vi "EF_ReadIniFile.vi"(11 "Path":path) -> (2 "EF_DAQThread_IniData":T1, 3 "EF_DAQThread_Data":T2)   [LabVIEW 2017]
uses:
  Types/EF_DAQThread_Data.ctl
  _lib/PQ/PicoHarp/PH_InitInfo.ctl
  Types/EF_GUIThread_IniData.ctl
  <vilib>/Utility/config.llb/Read Key (String).vi
  <vilib>/Utility/config.llb/Write Key (String).vi
  <vilib>/Utility/config.llb/Read Key (I32).vi
  <vilib>/Utility/config.llb/Write Key (I32).vi
  <vilib>/Utility/config.llb/Read Key (Double).vi
  <vilib>/Utility/config.llb/Write Key (Double).vi
  <vilib>/Utility/config.llb/Read Key (U32).vi
  <vilib>/Utility/config.llb/Write Key (U32).vi
  <vilib>/Utility/config.llb/NI_LVConfig.lvlib
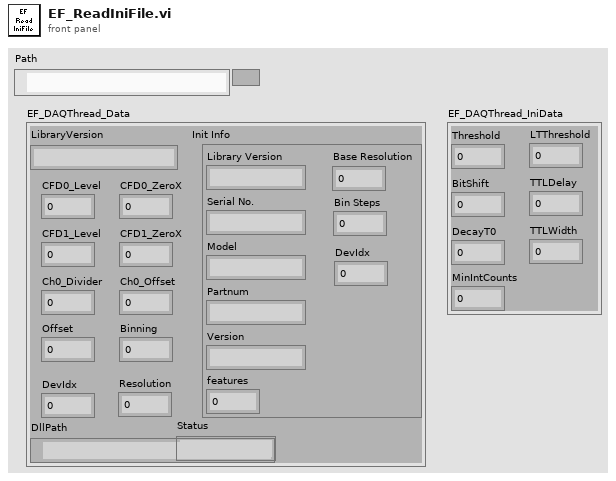
[diagram p1: front panel]
types:
  T1 = typedef "EF_GUIThread_IniData.ctl" = cluster{"Threshold":i32, "BitShift":i32, "DecayT0":dbl, "LTThreshold":dbl, "TTLDelay":i32, "TTLWidth":i32, "MinIntCounts":u32}
  T2 = typedef "EF_DAQThread_Data.ctl" = cluster{"LibraryVersion":string, "CFD0_Level":i32, "CFD0_ZeroX":i32, "CFD1_Level":i32, "CFD1_ZeroX":i32, "Ch0_Divider":i32, "Ch0_Offset":i32, "Init Info":T3, "DevIdx":i32, "Offset":i32, "Binning":i32, "Resolution":dbl, "DllPath":path, "Status":string}
  T3 = typedef "PH_InitInfo.ctl" = cluster{"Library Version":string, "Serial No.":string, "Model":string, "Partnum":string, "Version":string, "features":i32, "Base Resolution":dbl, "Bin Steps":i32, "DevIdx":i32}
  T4 = typedef "NI_LVConfig.lvlib/Config Data RefNum.ctl" = refnum<k1>
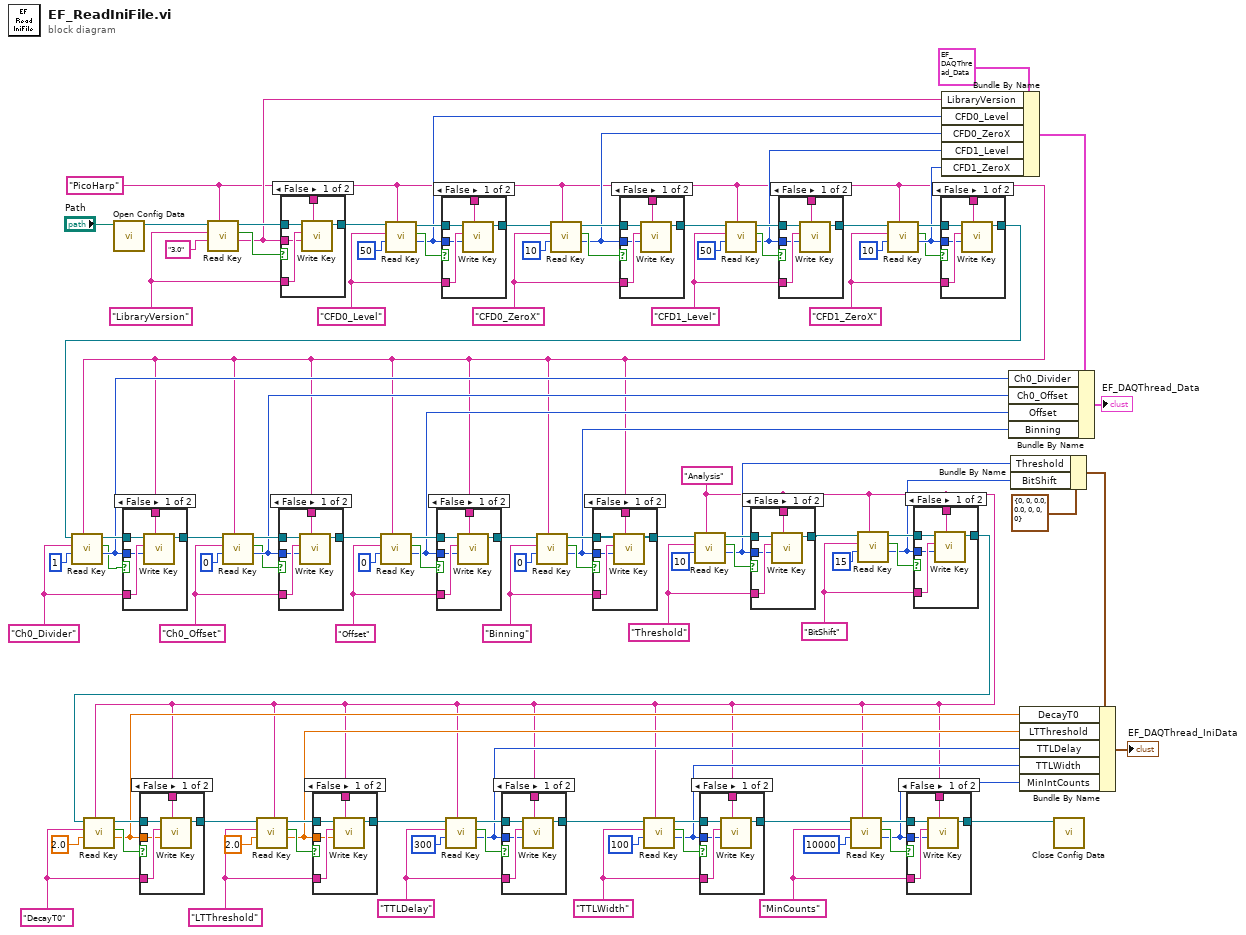
[diagram p0: block diagram]
diagram:
  w8 = "MinCounts" ("key")
  w19 = "TTLWidth" ("key")
  w27 = "TTLDelay" ("key")
  w29 = "LTThreshold" ("key")
  w37 = "DecayT0" ("key")
  w39 = "BitShift" ("key")
  w3 = "Analysis" ("section")
  w44 = "Threshold" ("key")
  w49 = "Binning" ("key")
  w55 = "Offset" ("key")
  w62 = "Ch0_Offset" ("key")
  w69 = "Ch0_Divider" ("key")
  w76 = "CFD1_ZeroX" ("key")
  w80 = "CFD1_Level" ("key")
  w83 = "CFD0_ZeroX" ("key")
  w89 = "CFD0_Level" ("key")
  w94 = "LibraryVersion" ("key")
  w48 = "PicoHarp" ("section")
  n1 = call <vilib>:"Open Config Data.vi"("configuration file path"="Path") -> ("refnum"=w105:T4)  [unwired: 8 in, 2 out]
  n2 = call-poly <vilib>:"Read Key.vi"("section"=w48, "default value"="3.0", "key"=w94, "refnum"=w105) -> ("value"=w93:string, "found?"=w96:bool, "refnum out"=w95:T4)  [unwired: 4 in, 1 out]
  n3 = case shown="False" w96 {
    tunnel: w95 -> [w111 w112]
    tunnel: w48 -> [w110 _]
    tunnel: w94 -> [w109 _]
    tunnel: w93 -> [w108 _]
    tunnel: [w107 w112] -> w92
    frame False {
      n4 = call-poly <vilib>:"Write Key.vi"("section"=w110, "value"=w108, "key"=w109, "refnum"=w111) -> ("refnum out"=w107:T4)  [unwired: 5 in, 2 out]
    }
    frame True {
    }
  }
  n5 = call-poly <vilib>:"Read Key.vi"("section"=w48, "default value"=50, "key"=w89, "refnum"=w92) -> ("value"=w88:i32, "found?"=w90:bool, "refnum out"=w91:T4)  [unwired: 4 in, 1 out]
  n6 = case shown="False" w90 {
    tunnel: w91 -> [w117 w118]
    tunnel: w48 -> [w116 _]
    tunnel: w89 -> [w115 _]
    tunnel: w88 -> [w114 _]
    tunnel: [w113 w118] -> w87
    frame False {
      n7 = call-poly <vilib>:"Write Key.vi"("section"=w116, "value"=w114, "key"=w115, "refnum"=w117) -> ("refnum out"=w113:T4)  [unwired: 5 in, 2 out]
    }
    frame True {
    }
  }
  n8 = call-poly <vilib>:"Read Key.vi"("section"=w48, "default value"=10, "key"=w83, "refnum"=w87) -> ("value"=w84:i32, "found?"=w85:bool, "refnum out"=w86:T4)  [unwired: 4 in, 1 out]
  n9 = case shown="False" w85 {
    tunnel: w86 -> [w123 w124]
    tunnel: w48 -> [w122 _]
    tunnel: w83 -> [w121 _]
    tunnel: w84 -> [w120 _]
    tunnel: [w119 w124] -> w82
    frame False {
      n10 = call-poly <vilib>:"Write Key.vi"("section"=w122, "value"=w120, "key"=w121, "refnum"=w123) -> ("refnum out"=w119:T4)  [unwired: 5 in, 2 out]
    }
    frame True {
    }
  }
  n11 = call-poly <vilib>:"Read Key.vi"("section"=w48, "default value"=50, "key"=w80, "refnum"=w82) -> ("value"=w78:i32, "found?"=w79:bool, "refnum out"=w81:T4)  [unwired: 4 in, 1 out]
  n12 = case shown="False" w79 {
    tunnel: w81 -> [w129 w130]
    tunnel: w48 -> [w128 _]
    tunnel: w80 -> [w127 _]
    tunnel: w78 -> [w126 _]
    tunnel: [w125 w130] -> w61
    frame False {
      n13 = call-poly <vilib>:"Write Key.vi"("section"=w128, "value"=w126, "key"=w127, "refnum"=w129) -> ("refnum out"=w125:T4)  [unwired: 5 in, 2 out]
    }
    frame True {
    }
  }
  n14 = call-poly <vilib>:"Read Key.vi"("section"=w48, "default value"=10, "key"=w76, "refnum"=w61) -> ("value"=w75:i32, "found?"=w74:bool, "refnum out"=w77:T4)  [unwired: 4 in, 1 out]
  n15 = case shown="False" w74 {
    tunnel: w77 -> [w135 w136]
    tunnel: w48 -> [w134 _]
    tunnel: w76 -> [w133 _]
    tunnel: w75 -> [w132 _]
    tunnel: [w131 w136] -> w73
    frame False {
      n16 = call-poly <vilib>:"Write Key.vi"("section"=w134, "value"=w132, "key"=w133, "refnum"=w135) -> ("refnum out"=w131:T4)  [unwired: 5 in, 2 out]
    }
    frame True {
    }
  }
  n17 = call-poly <vilib>:"Read Key.vi"("section"=w48, "default value"=1, "key"=w69, "refnum"=w73) -> ("value"=w68:i32, "found?"=w67:bool, "refnum out"=w70:T4)  [unwired: 4 in, 1 out]
  n18 = case shown="False" w67 {
    tunnel: w70 -> [w141 w142]
    tunnel: w48 -> [w140 _]
    tunnel: w69 -> [w139 _]
    tunnel: w68 -> [w138 _]
    tunnel: [w137 w142] -> w66
    frame False {
      n19 = call-poly <vilib>:"Write Key.vi"("section"=w140, "value"=w138, "key"=w139, "refnum"=w141) -> ("refnum out"=w137:T4)  [unwired: 5 in, 2 out]
    }
    frame True {
    }
  }
  n20 = call-poly <vilib>:"Read Key.vi"("section"=w48, "default value"=0, "key"=w62, "refnum"=w66) -> ("value"=w64:i32, "found?"=w63:bool, "refnum out"=w65:T4)  [unwired: 4 in, 1 out]
  n21 = case shown="False" w63 {
    tunnel: w65 -> [w147 w148]
    tunnel: w48 -> [w146 _]
    tunnel: w62 -> [w145 _]
    tunnel: w64 -> [w144 _]
    tunnel: [w143 w148] -> w57
    frame False {
      n22 = call-poly <vilib>:"Write Key.vi"("section"=w146, "value"=w144, "key"=w145, "refnum"=w147) -> ("refnum out"=w143:T4)  [unwired: 5 in, 2 out]
    }
    frame True {
    }
  }
  n23 = call-poly <vilib>:"Read Key.vi"("section"=w48, "default value"=0, "key"=w55, "refnum"=w57) -> ("value"=w56:i32, "found?"=w60:bool, "refnum out"=w59:T4)  [unwired: 4 in, 1 out]
  n24 = case shown="False" w60 {
    tunnel: w59 -> [w153 w154]
    tunnel: w48 -> [w152 _]
    tunnel: w55 -> [w151 _]
    tunnel: w56 -> [w150 _]
    tunnel: [w149 w154] -> w51
    frame False {
      n25 = call-poly <vilib>:"Write Key.vi"("section"=w152, "value"=w150, "key"=w151, "refnum"=w153) -> ("refnum out"=w149:T4)  [unwired: 5 in, 2 out]
    }
    frame True {
    }
  }
  n26 = call-poly <vilib>:"Read Key.vi"("section"=w48, "default value"=0, "key"=w49, "refnum"=w51) -> ("value"=w50:i32, "found?"=w52:bool, "refnum out"=w53:T4)  [unwired: 4 in, 1 out]
  n27 = case shown="False" w52 {
    tunnel: w53 -> [w159 w160]
    tunnel: w48 -> [w158 _]
    tunnel: w49 -> [w157 _]
    tunnel: w50 -> [w156 _]
    tunnel: [w155 w160] -> w38
    frame False {
      n28 = call-poly <vilib>:"Write Key.vi"("section"=w158, "value"=w156, "key"=w157, "refnum"=w159) -> ("refnum out"=w155:T4)  [unwired: 5 in, 2 out]
    }
    frame True {
    }
  }
  n29 = call-poly <vilib>:"Read Key.vi"("section"=w3, "default value"=10, "key"=w44, "refnum"=w38) -> ("value"=w16:i32, "found?"=w45:bool, "refnum out"=w46:T4)  [unwired: 4 in, 1 out]
  n30 = case shown="False" w45 {
    tunnel: w46 -> [w165 w166]
    tunnel: w3 -> [w164 _]
    tunnel: w44 -> [w163 _]
    tunnel: w16 -> [w162 _]
    tunnel: [w161 w166] -> w40
    frame False {
      n31 = call-poly <vilib>:"Write Key.vi"("section"=w164, "value"=w162, "key"=w163, "refnum"=w165) -> ("refnum out"=w161:T4)  [unwired: 5 in, 2 out]
    }
    frame True {
    }
  }
  n32 = call-poly <vilib>:"Read Key.vi"("section"=w3, "default value"=15, "key"=w39, "refnum"=w40) -> ("value"=w15:i32, "found?"=w43:bool, "refnum out"=w42:T4)  [unwired: 4 in, 1 out]
  n33 = case shown="False" w43 {
    tunnel: w42 -> [w171 w172]
    tunnel: w3 -> [w170 _]
    tunnel: w39 -> [w169 _]
    tunnel: w15 -> [w168 _]
    tunnel: [w167 w172] -> w33
    frame False {
      n34 = call-poly <vilib>:"Write Key.vi"("section"=w170, "value"=w168, "key"=w169, "refnum"=w171) -> ("refnum out"=w167:T4)  [unwired: 5 in, 2 out]
    }
    frame True {
    }
  }
  n35 = call-poly <vilib>:"Read Key.vi"("section"=w3, "default value"=2.0, "key"=w37, "refnum"=w33) -> ("value"=w13:dbl, "found?"=w34:bool, "refnum out"=w35:T4)  [unwired: 4 in, 1 out]
  n36 = case shown="False" w34 {
    tunnel: w35 -> [w177 w178]
    tunnel: w3 -> [w176 _]
    tunnel: w37 -> [w175 _]
    tunnel: w13 -> [w174 _]
    tunnel: [w173 w178] -> w28
    frame False {
      n37 = call-poly <vilib>:"Write Key.vi"("section"=w176, "value"=w174, "key"=w175, "refnum"=w177) -> ("refnum out"=w173:T4)  [unwired: 5 in, 2 out]
    }
    frame True {
    }
  }
  n38 = call-poly <vilib>:"Read Key.vi"("section"=w3, "default value"=2.0, "key"=w29, "refnum"=w28) -> ("value"=w12:dbl, "found?"=w32:bool, "refnum out"=w31:T4)  [unwired: 4 in, 1 out]
  n39 = case shown="False" w32 {
    tunnel: w31 -> [w183 w184]
    tunnel: w3 -> [w182 _]
    tunnel: w29 -> [w181 _]
    tunnel: w12 -> [w180 _]
    tunnel: [w179 w184] -> w23
    frame False {
      n40 = call-poly <vilib>:"Write Key.vi"("section"=w182, "value"=w180, "key"=w181, "refnum"=w183) -> ("refnum out"=w179:T4)  [unwired: 5 in, 2 out]
    }
    frame True {
    }
  }
  n41 = call-poly <vilib>:"Read Key.vi"("section"=w3, "default value"=300, "key"=w27, "refnum"=w23) -> ("value"=w11:i32, "found?"=w24:bool, "refnum out"=w25:T4)  [unwired: 4 in, 1 out]
  n42 = case shown="False" w24 {
    tunnel: w25 -> [w189 w190]
    tunnel: w3 -> [w188 _]
    tunnel: w27 -> [w187 _]
    tunnel: w11 -> [w186 _]
    tunnel: [w185 w190] -> w18
    frame False {
      n43 = call-poly <vilib>:"Write Key.vi"("section"=w188, "value"=w186, "key"=w187, "refnum"=w189) -> ("refnum out"=w185:T4)  [unwired: 5 in, 2 out]
    }
    frame True {
    }
  }
  n44 = call-poly <vilib>:"Read Key.vi"("section"=w3, "default value"=100, "key"=w19, "refnum"=w18) -> ("value"=w10:i32, "found?"=w22:bool, "refnum out"=w21:T4)  [unwired: 4 in, 1 out]
  n45 = case shown="False" w22 {
    tunnel: w21 -> [w195 w196]
    tunnel: w3 -> [w194 _]
    tunnel: w19 -> [w193 _]
    tunnel: w10 -> [w192 _]
    tunnel: [w191 w196] -> w4
    frame False {
      n46 = call-poly <vilib>:"Write Key.vi"("section"=w194, "value"=w192, "key"=w193, "refnum"=w195) -> ("refnum out"=w191:T4)  [unwired: 5 in, 2 out]
    }
    frame True {
    }
  }
  n47 = call-poly <vilib>:"Read Key.vi"("section"=w3, "default value"=u32 10000, "key"=w8, "refnum"=w4) -> ("value"=w1:u32, "found?"=w5:bool, "refnum out"=w6:T4)  [unwired: 4 in, 1 out]
  n48 = case shown="False" w5 {
    tunnel: w6 -> [w201 w202]
    tunnel: w3 -> [w200 _]
    tunnel: w8 -> [w199 _]
    tunnel: w1 -> [w198 _]
    tunnel: [w197 w202] -> w2
    frame False {
      n49 = call-poly <vilib>:"Write Key.vi"("section"=w200, "value"=w198, "key"=w199, "refnum"=w201) -> ("refnum out"=w197:T4)  [unwired: 5 in, 2 out]
    }
    frame True {
    }
  }
  n50 = Bundle By Name(cluster=T2 {"LibraryVersion"="", "CFD0_Level"=0, "CFD0_ZeroX"=0, "CFD1_Level"=0, "CFD1_ZeroX"=0, "Ch0_Divider"=0, "Ch0_Offset"=0, "Init Info"={"Library Version"="", "Serial No."="", "Model"="", "Partnum"="", "Version"="", "features"=0, "Base Resolution"=0.0, "Bin Steps"=0, "DevIdx"=0}, "DevIdx"=0, "Offset"=0, "Binning"=0, "Resolution"=0.0, "DllPath"=path "", "Status"=""} ("EF_DAQThread_Data_in"), "LibraryVersion"=w93, "CFD0_Level"=w88, "CFD0_ZeroX"=w84, "CFD1_Level"=w78, "CFD1_ZeroX"=w75) -> (w72:T2)
  n51 = Bundle By Name(cluster=w72, "Ch0_Divider"=w68, "Ch0_Offset"=w64, "Offset"=w56, "Binning"=w50) -> (→"EF_DAQThread_Data":T2)
  n52 = Bundle By Name(cluster=T1 {"Threshold"=0, "BitShift"=0, "DecayT0"=0.0, "LTThreshold"=0.0, "TTLDelay"=0, "TTLWidth"=0, "MinIntCounts"=0} ("EF_GUIThread_IniData"), "Threshold"=w16, "BitShift"=w15) -> (w14:T1)
  n53 = Bundle By Name(cluster=w14, "DecayT0"=w13, "LTThreshold"=w12, "TTLDelay"=w11, "TTLWidth"=w10, "MinIntCounts"=w1) -> (→"EF_DAQThread_IniData":T1)
  n54 = call <vilib>:"Close Config Data.vi"("refnum"=w2) -> ()  [unwired: 9 in, 2 out]
